vi "Grid_MLS_point.vi"(10 "MultiLineSegment Array":T1(array[cluster])) -> (2 "points":i32)   [LabVIEW 2021]
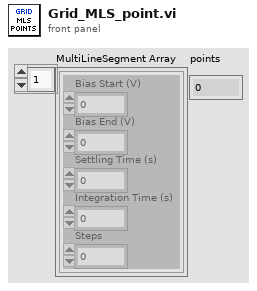
[diagram p1: front panel]
types:
  T1 = cluster{"Bias Start (V)":sgl, "Bias End (V)":sgl, "Settling Time (s)":sgl, "Integration Time (s)":sgl, "Steps":sgl}[]
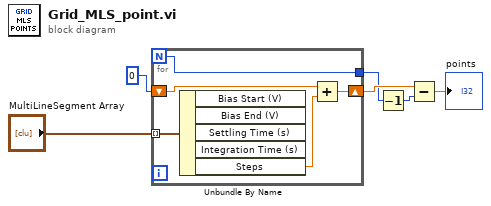
[diagram p0: block diagram]
diagram:
  n1 = for {
    N -> [w7]
    tunnel: "MultiLineSegment Array" -> [w11] mode=indexing
    shift-right: [w9] -> w6
    shift-left: 0 -> [w8]
    tunnel: [w7] -> w5
    n2 = Unbundle By Name(w11) -> ("Steps"=w10:sgl)  [unwired: 4 out]
    n3 = Add(x=w8, y=w10) -> (x+y=w9:sgl)
  }
  n4 = Decrement(x=w5) -> (x-1=w4:i32)
  n5 = Subtract(x=w6, y=w4) -> (x-y=→"points":sgl)
